vi "Connet_Callback.vi"(4 "사용자 파라미터":variant, 5 "이벤트 데이터":cluster{"nErrCode":i32}, 6 "컨트롤 참조":refnum<k7>, 7 "이벤트 일반 데이터":cluster{"이벤트 소스":i32, "이벤트 타입":u32, "타임스탬프":u32}) -> ()   [LabVIEW 2018]
uses:
  Global Value.vi
panel:
  out "불리언":bool
  out "접속 문자열":string
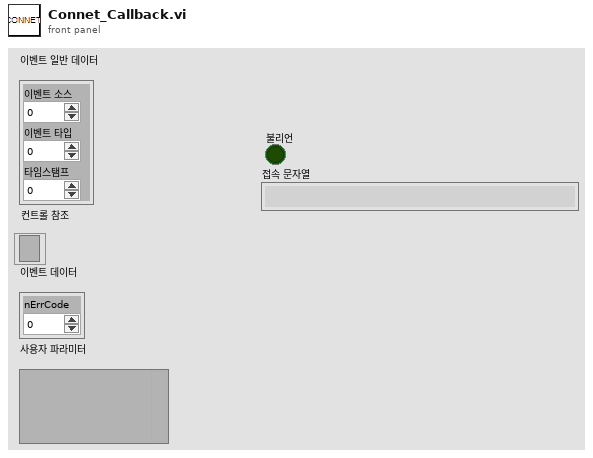
[diagram p1: front panel]
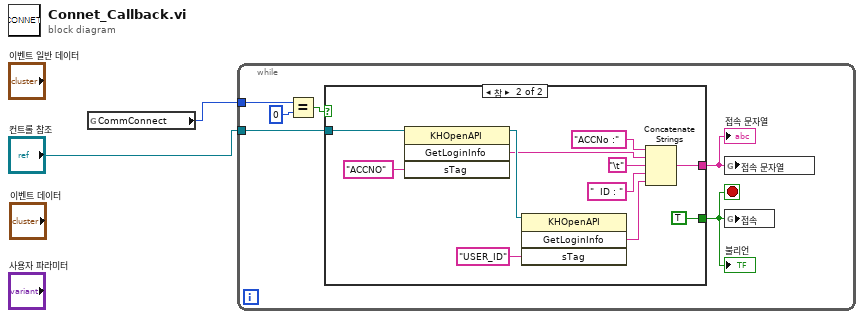
[diagram p0: block diagram]
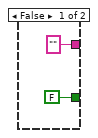
[diagram p2: hidden frame]
diagram:
  n1 = global read "Global Value.vi" "CommConnect"() -> (w1:i32)
  n2 = while {
    tunnel: "컨트롤 참조" -> [w6]
    tunnel: w1 -> [w5]
    stop <- w4 stop-if-true
    n3 = Equal?(x=w5, y=0) -> (x = y?=w7:bool)
    n4 = case shown="참" w7 {
      tunnel: ["" w21] -> w3
      tunnel: w6 -> [_ w20]
      tunnel: [FALSE TRUE] -> w4
      frame False {
      }
      frame True {
        n5 = invoke class="KHOpenAPI" method="GetLoginInfo"(reference=w20, "sTag"="ACCNO") -> (reference out=w17:refnum<k7>, "GetLoginInfo"=w16:string)  [unwired: 2 in, 2 out]
        n6 = invoke class="KHOpenAPI" method="GetLoginInfo"(reference=w17, "sTag"="USER_ID") -> ("GetLoginInfo"=w13:string)  [unwired: 2 in, 3 out]
        n7 = Concatenate Strings("ACCNo :" ("문자열"), w16, "\t", "  ID : " ("문자열"), w13) -> (w21:string)
      }
    }
    "접속 문자열" <- w3
    "불리언" <- w4
    n8 = global write "Global Value.vi" "접속 문자열"(w3) -> ()
    n9 = global write "Global Value.vi" "접속"(w4) -> ()
  }
